vi "build_waveform.vi"(10 "Off times":i32[](array[numeric]), 11 "On times":i32[](array[numeric])) -> (2 "max time":i32, 3 "Output":u8[](array[numeric]))   [LabVIEW 2012]
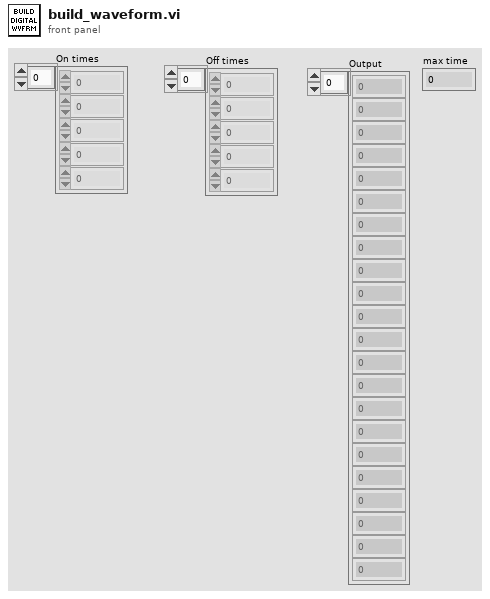
[diagram p1: front panel]
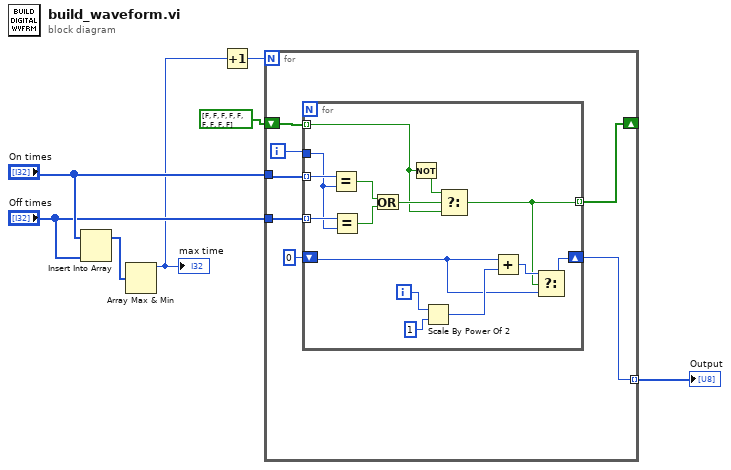
[diagram p0: block diagram]
diagram:
  n1 = Insert Into Array(array="On times", new element="Off times") -> (w5:i32[])  [unwired: 1 in]
  n2 = Array Max & Min(array=w5) -> (max value=w1:i32)  [unwired: 3 out]
  "max time" <- w1
  n3 = Increment(x=w1) -> (x+1=w2:i32)
  n4 = for {
    N: w2 -> [_]
    shift-right: [w12] -> _
    shift-left: bool[] [FALSE, FALSE, FALSE, FALSE, FALSE, FALSE, FALSE, FALSE, FALSE] -> [w11]
    tunnel: "On times" -> [w14]
    tunnel: "Off times" -> [w13]
    tunnel: [w9] -> w6 mode=indexing
    i -> [w8]
    n5 = for {
      tunnel: w14 -> [w29] mode=indexing
      tunnel: w13 -> [w28] mode=indexing
      tunnel: w8 -> [w27]
      tunnel: [w17] -> w12 mode=indexing
      tunnel: w11 -> [w22] mode=indexing
      shift-right: [w15] -> w9
      shift-left: u8 0 ("x") -> [w16]
      i -> [w18]
      n6 = Equal?(x=w29, y=w27) -> (x = y?=w25:bool)
      n7 = Equal?(x=w28, y=w27) -> (x = y?=w26:bool)
      n8 = Or(x=w25, y=w26) -> (x .or. y?=w24:bool)
      n9 = Not(x=w22) -> (.not. x?=w23:bool)
      n10 = Scale By Power Of 2(n=w18, x=u8 1) -> (x*2^n=w21:u8)
      n11 = Select(t=w23, s=w24, f=w22) -> (s? t:f=w17:bool)
      n12 = Add(x=w16, y=w21) -> (x+y=w19:u8)
      n13 = Select(t=w19, s=w17, f=w16) -> (s? t:f=w15:u8)
    }
  }
  "Output" <- w6
